vi "Get References.vi"(8 "error in (no error)":errorcluster, 11 "MCListbox with Checkboxes in":refnum<class "MCListbox with Checkboxes.lvclass">) -> (0 "error out":errorcluster, 1 "Check All":refnum<vi>, 2 "Multicolumn Listbox":refnum<vi>, 3 "MCListbox with Checkboxes out":refnum<class "MCListbox with Checkboxes.lvclass">)   [LabVIEW 2016, in "MCListbox with Checkboxes.lvclass"]
uses:
  MCListbox with Checkboxes.lvclass
  MCListbox with Checkboxes.lvclass/MCListbox with Checkboxes.ctl
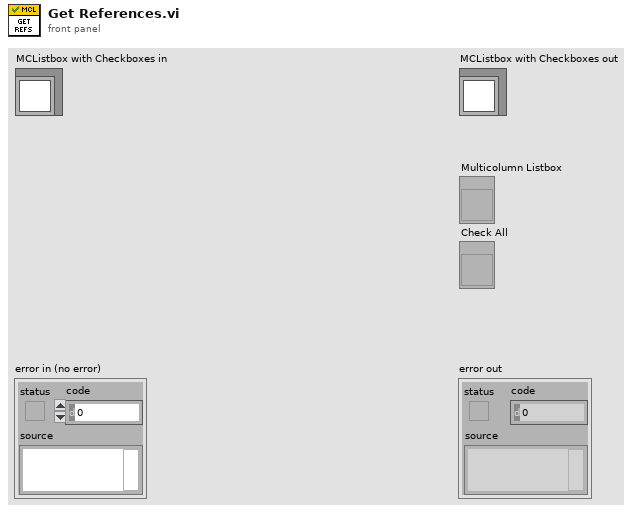
[diagram p1: front panel]
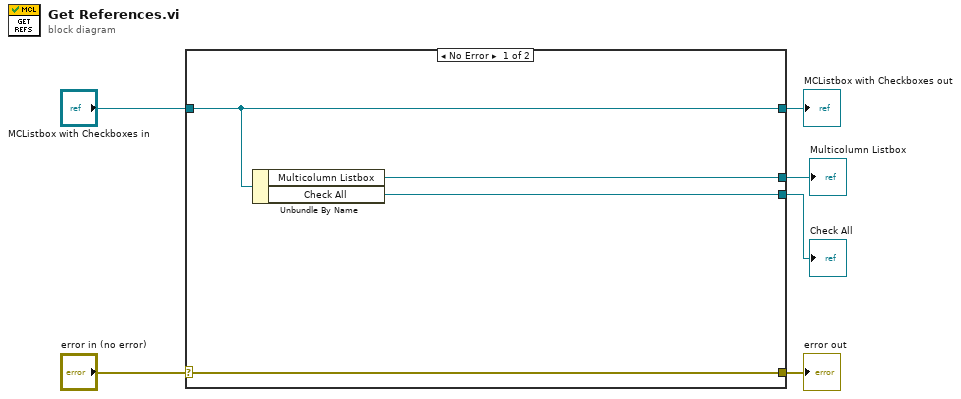
[diagram p0: block diagram]
diagram:
  n1 = case shown="No Error" "error in (no error)" {
    selector: "error in (no error)" -> [w10 w12]
    tunnel: [w10 w12] -> w5
    tunnel: [w9 w11] -> w3
    tunnel: "MCListbox with Checkboxes in" -> [w9 w11]
    tunnel: [w8 _] -> w2
    tunnel: [w7 _] -> w1
    frame No Error {
      n2 = Unbundle By Name(w9) -> ("Multicolumn Listbox"=w8:refnum<vi>, "Check All"=w7:refnum<vi>)
    }
    frame Error {
    }
  }
  "error out" <- w5
  "MCListbox with Checkboxes out" <- w3
  "Multicolumn Listbox" <- w2
  "Check All" <- w1
